vi "Get Threats (SubVI).vi"(0 "pathConfigIN":path, 2 "refThreat":refnum<vi>, 3 "error in":errorcluster) -> (5 "stringOut":string[](array[string]), 6 "pathConfigOUT":path, 8 "factorOut":sgl[](array[numeric]), 9 "error out":errorcluster)   [LabVIEW 2015]
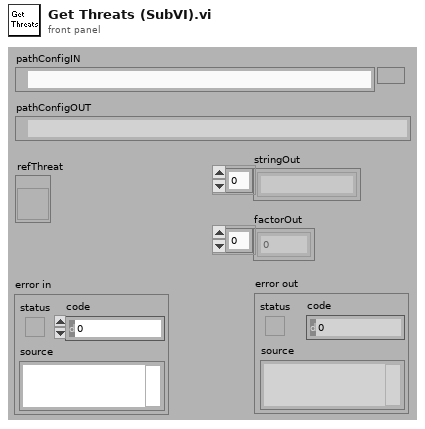
[diagram p1: front panel]
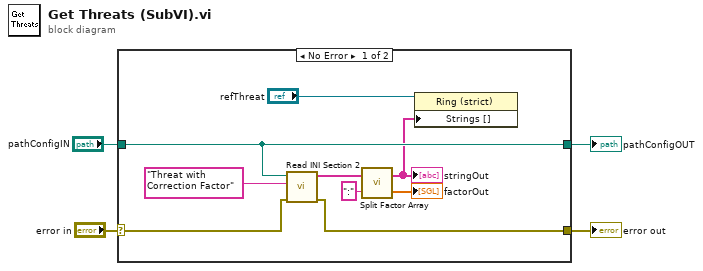
[diagram p0: block diagram]
diagram:
  n1 = case shown="No Error" "error in" {
    selector: "error in" -> [w9 w15]
    tunnel: [w8 w15] -> w3
    tunnel: "pathConfigIN" -> [w7 w14]
    tunnel: [w7 w14] -> w1
    frame No Error {
      n2 = call "Read INI Section 2.vi"("error IN"=w9, "section"="Threat with Correction Factor", "configuration file path"=w7) -> ("error OUT"=w8:errorcluster, "Array"=w11:string[])  [unwired: 1 in, 2 out]
      n3 = call "Split Factor Array.vi"("Split character"=":", "STRING INPUT"=w11) -> ("FACTOR OUTPUT"=→"factorOut":sgl[], "STRING OUTPUT"=w5:string[])
      "stringOut" <- w5
      n4 = property class="Ring (strict)"(reference="refThreat", "Strings []"=w5) -> ()  [unwired: 1 in, 2 out]
    }
    frame Error {
    }
  }
  "error out" <- w3
  "pathConfigOUT" <- w1
